vi "Shooter Set PID.vi"(10 "RPM Target":dbl, 11 "CAN Talon SRX Ref In":T1={"DeviceStatus"={"status"=FALSE, "code"=0, "source"=""}, "Type"=enum."PWM", "PWM"={"PWM Channel"=enum."PWM 1", "DeadBand"={"Name"="", "maxPositivePwm"=0, "minPositivePwm"=0, "centerPwm"=0, "maxNegativePwm"=0, "minNegativePwm"=0, "angularRange"=0}}, "CAN"={"Device Number"=0, "SetOutput VI Ref"=variant(enum8{"Percent VBus", "Current", "Speed", "Position", "Voltage"} enum."Percent VBus"), "GetOutput VI Ref"=variant(refnum<k1> refnum), "Enable VI Ref"=variant(dbl 12.0), "Disable VI Ref"=variant(enum8{"Percent VBus", "Speed", "Position", "Slave", "Unchanged / Invalid", "Voltage Compensation", "Current", "Motion Profile"} enum."Percent VBus"), "Data"=variant}, "Invert"=FALSE}) -> (3 "CAN Talon SRX Ref Out":T1={"DeviceStatus"={"status"=FALSE, "code"=0, "source"=""}, "Type"=enum."PWM", "PWM"={"PWM Channel"=enum."PWM 1", "DeadBand"={"Name"="", "maxPositivePwm"=0, "minPositivePwm"=0, "centerPwm"=0, "maxNegativePwm"=0, "minNegativePwm"=0, "angularRange"=0}}, "CAN"={"Device Number"=0, "SetOutput VI Ref"=variant(enum8{"Percent VBus", "Current", "Speed", "Position", "Voltage"} enum."Percent VBus"), "GetOutput VI Ref"=variant(refnum<k1> refnum), "Enable VI Ref"=variant(dbl 12.0), "Disable VI Ref"=variant(enum8{"Percent VBus", "Speed", "Position", "Slave", "Unchanged / Invalid", "Voltage Compensation", "Current", "Motion Profile"} enum."Percent VBus"), "Data"=variant}, "Invert"=FALSE})   [LabVIEW 2016]
uses:
  <vilib>/Rock Robotics/WPI/MotorControl/WPI_MotorControlDeviceRef.ctl
  <vilib>/Rock Robotics/WPI/MotorControl/WPI_MotorControlType.ctl
  <vilib>/Rock Robotics/SystemInterfaces/DIO/FPGA_DIOPWMChannel.ctl
  <vilib>/Rock Robotics/WPI/PWM/WPI_PWMDeadband.ctl
  <vilib>/Rock Robotics/WPI/ThirdParty/CanMotor/TalonSRX/WPI_CANTalonSRX_APIControlMode.ctl
  Robot Global Data.vi
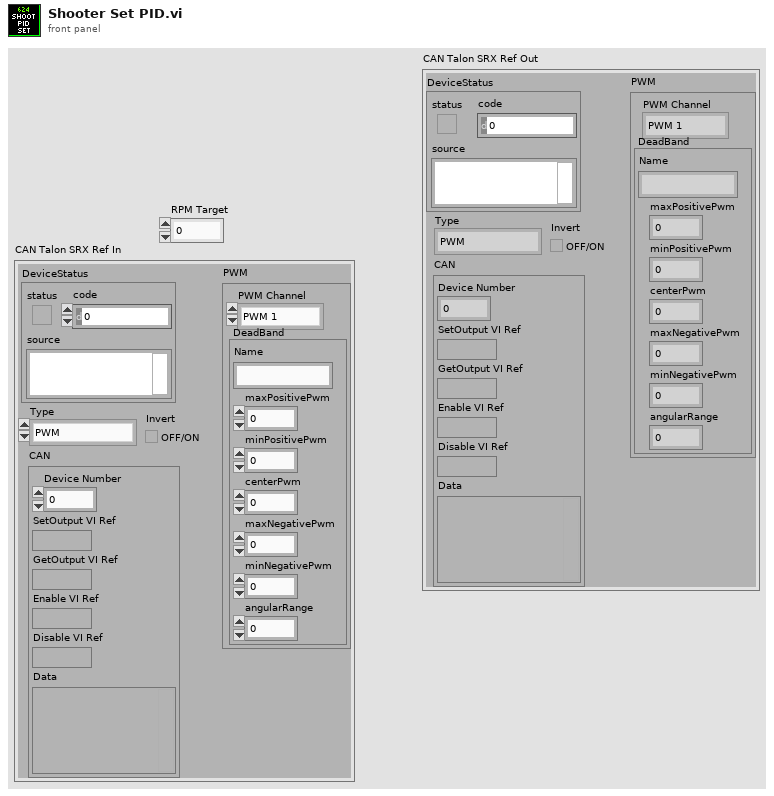
[diagram p1: front panel]
types:
  T1 = typedef "WPI_MotorControlDeviceRef.ctl" = cluster{"DeviceStatus":errorcluster, "Type":T2, "PWM":cluster{"PWM Channel":T3, "DeadBand":T4}, "CAN":cluster{"Device Number":u8, "SetOutput VI Ref":variant, "GetOutput VI Ref":variant, "Enable VI Ref":variant, "Disable VI Ref":variant, "Data":variant}, "Invert":bool}
  T2 = typedef "WPI_MotorControlType.ctl" = enum16{"PWM", "CAN"}
  T3 = typedef "FPGA_DIOPWMChannel.ctl" = enum8{"PWM 0", "PWM 1", "PWM 2", "PWM 3", "PWM 4", "PWM 5", "PWM 6", "PWM 7", "PWM 8", "PWM 9", "PWM MXP 0", "PWM MXP 1", "PWM MXP 2", "PWM MXP 3", "PWM MXP 4", "PWM MXP 5", "PWM MXP 6", "PWM MXP 7", "PWM MXP 8", "PWM MXP 9", "Invalid"}
  T4 = typedef "WPI_PWMDeadband.ctl" = cluster{"Name":string, "maxPositivePwm":i32, "minPositivePwm":i32, "centerPwm":i32, "maxNegativePwm":i32, "minNegativePwm":i32, "angularRange":u16}
  T5 = typedef "Dashboard Control Data.ctl" = cluster{"Drivetrain Settings":T6, "Intake Presets ":T8, "Shooter Presets":T9, "Vision Target Packet":T10, "Auton Presets":cluster{"Start Position":dbl}, "Drivetrain Encoder Values":T11, "Drivetrain Encoder Settings":cluster{"Left Tick Constant":dbl, "Right Tick Contant":dbl, "Reset Encoders":bool, "Center Tick Constant":dbl}, "Zero Gyro":bool, "Vision Timeout":dbl}
  T6 = typedef "Drivetrain Settings.ctl" = cluster{"Gyro Tolerance":dbl, "Gyro Steer PID Gains":T7, "Y Power Multiplier":dbl, "Turn Power Multiplier":dbl, "Gyro Output":dbl, "Creep Rate":dbl, "Distance Drive PID Gains":T7, "Distance Tolerance":dbl, "Distance Output":dbl, "Strafe Threshold":dbl, "Strafe Correct":bool, "Strafe Corect Tolerance":dbl, "Translate Drive PID Gains":T7, "Strafe Output":dbl, "SC Right":dbl, "SC Left":dbl, "Use Gyro":bool, "Constant Power":bool, "Strafe Power":dbl}
  T7 = typedef "PID Gains.ctl" = cluster{"proportional gain (Kc)":dbl, "integral time (Ti, min)":dbl, "derivative time (Td, min)":dbl}
  T8 = typedef "Intake Presets.ctl" = cluster{"Intake Speed ":dbl, "Outake Speed":dbl, "Current Trip Delay":dbl, "Max Current":dbl}
  T9 = typedef "Shooter Presets.ctl" = cluster{"Key Shot":cluster{"RPM ":dbl, "Hood?":bool}, "Distance Shot":cluster{"RPM":dbl, "Hood?":bool}, "RPM Tolerance":dbl, "Unstuck Delay Time ":dbl, "Initial RPM Increase":dbl, "Warmup Delay":dbl, "Faster Time":dbl, "Shooter PID Gains":cluster{"P":dbl, "I":dbl, "D":dbl, "FF":dbl, "Ramp Rate":dbl, "I Zone":dbl}}
  T10 = typedef "Vision Target Packet.ctl" = cluster{"Robot Center":dbl, "Center X":dbl, "Center Y":dbl, "Angle":dbl, "Distance":dbl, "Found Target?":bool}
  T11 = typedef "Drivetrain Encoder Values.ctl" = cluster{"Left Encoder":T12, "Center Encoder":T12, "Right Encoder":T12}
  T12 = typedef "Encoder Values.ctl" = cluster{"Distance":dbl, "Speed":dbl, "Tick":dbl}
  T13 = typedef "WPI_CANTalonSRX_APIControlMode.ctl" = enum8{"Percent VBus", "Speed", "Position", "Slave", "Unchanged / Invalid", "Voltage Compensation", "Current", "Motion Profile", "Motion Magic"}
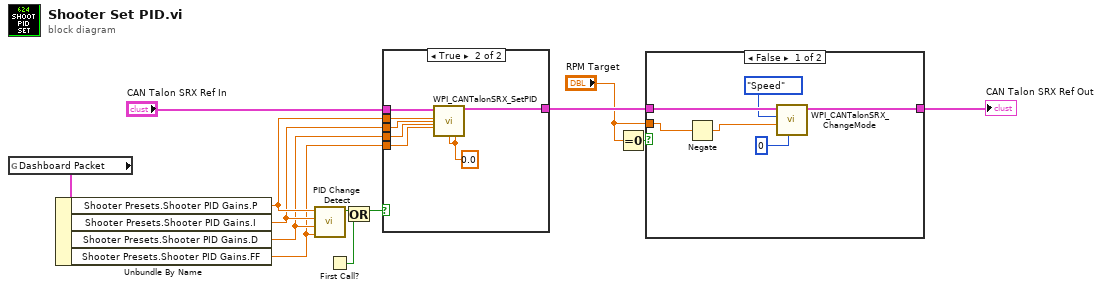
[diagram p0: block diagram]
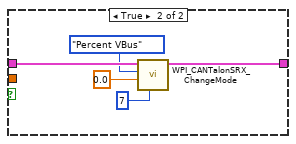
[diagram p2: hidden frame]
diagram:
  n1 = global read "Robot Global Data.vi" "Dashboard Packet"() -> (w12:T5)
  n2 = Unbundle By Name(w12) -> ("Shooter Presets.Shooter PID Gains.P"=w11:dbl, "Shooter Presets.Shooter PID Gains.I"=w10:dbl, "Shooter Presets.Shooter PID Gains.D"=w9:dbl, "Shooter Presets.Shooter PID Gains.FF"=w8:dbl)
  n3 = call "PID Change Detect.vi"("FF"=w8, "D"=w9, "I"=w10, "P"=w11) -> ("Changed?"=w7:bool)  [unwired: 7 in]
  n4 = First Call?() -> (First Call?: T/F=w1:bool)
  n5 = Or(x=w7, y=w1) -> (x .or. y?=w2:bool)
  n6 = case shown="True" w2 {
    tunnel: "CAN Talon SRX Ref In" -> [w14 w21]
    tunnel: [w14 w20] -> w6
    tunnel: w11 -> [_ w19]
    tunnel: w10 -> [_ w18]
    tunnel: w9 -> [_ w17]
    tunnel: w8 -> [_ w16]
    frame False {
    }
    frame True {
      w15 = 0.0 ("Ramp Rate")
      n7 = call <vilib>:"WPI_CANTalonSRX_SetPID.vi"("CAN Talon SRX Ref"=w21, "P"=w19, "I"=w18, "D"=w17, "F"=w16, "I Zone"=w15, "Ramp Rate"=w15) -> ("CAN Talon SRX Ref"=w20:T1)  [unwired: 7 in, 1 out]
    }
  }
  n8 = Equal To 0?(x="RPM Target") -> (x = 0?=w4:bool)
  n9 = case shown="False" w4 {
    tunnel: w6 -> [w27 w32]
    tunnel: "RPM Target" -> [w23 _]
    tunnel: [w26 w31] -> w3
    frame False {
      n10 = Negate(x=w23) -> (-x=w22:dbl)
      n11 = call <vilib>:"WPI_CANTalonSRX_ChangeMode.vi"("Master Device Number"=u8 0, "Output"=w22, "Control Mode"=WPI_CANTalonSRX_APIControlMode."Speed", "CAN Talon SRX Ref"=w27) -> ("CAN Talon SRX Ref"=w26:T1)  [unwired: 6 in, 1 out]
    }
    frame True {
      n12 = call <vilib>:"WPI_CANTalonSRX_ChangeMode.vi"("Master Device Number"=u8 7, "Output"=0.0, "Control Mode"=WPI_CANTalonSRX_APIControlMode."Percent VBus", "CAN Talon SRX Ref"=w32) -> ("CAN Talon SRX Ref"=w31:T1)  [unwired: 6 in, 1 out]
    }
  }
  "CAN Talon SRX Ref Out" <- w3
